vi "Write to Machine .vi"(8 "error in (no error)":errorcluster, 10 "G-Code String In":string, 11 "Machine In":refnum<visa-resource-name>) -> (0 "error out":errorcluster, 3 "Machine Out":refnum<visa-resource-name>)   [LabVIEW 2017]
doc: "Sends command (string) to machine.\n\n<B>Inputs</B>: \n- Machine In: Specifies the desired machine connected to computer via USB.\n- G-Code String In: Sends string command to machine. \n- Error In: Reads error (if any) from previous vi. \n\n<B>Outputs</B>: \n- Machine Out: Reference to the selected USB device.\n- Error Out: Returns an error if one occurs in vi (or has occurred in a previous vi), and passes it to next wired terminal."
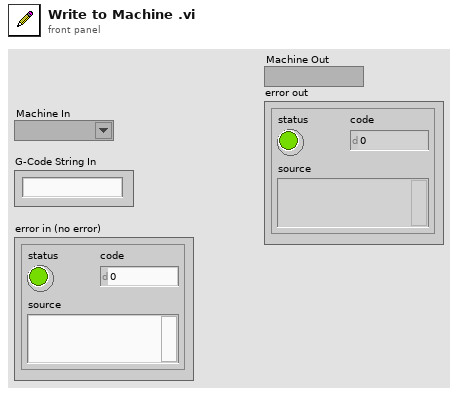
[diagram p1: front panel]
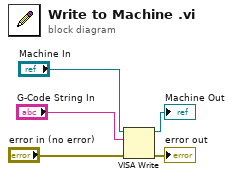
[diagram p0: block diagram]
diagram:
  n1 = VISA Write(VISA resource name="Machine In", write buffer="G-Code String In", error in (no error)="error in (no error)") -> (VISA resource name out=→"Machine Out":refnum<visa-resource-name>, error out=→"error out":errorcluster)  [unwired: 1 out]
